vi "3a - QDSM message.vi"() -> ()   [LabVIEW 2015]
uses:
  State/Parent Actor.lvclass
  Child Actor/Child Actor.lvclass
panel:
  in  "Choose Actor":bool
  out "On Off Indicator":bool
  out "Dirrection indicator":enum16{"Forward", "Reverse"}(ring)
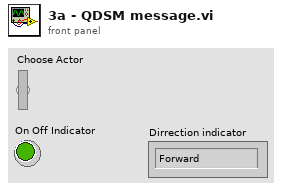
[diagram p1: front panel]
types:
  T1 = cluster{"Command":string, "Data":enum16{"Forward", "Reverse"}}
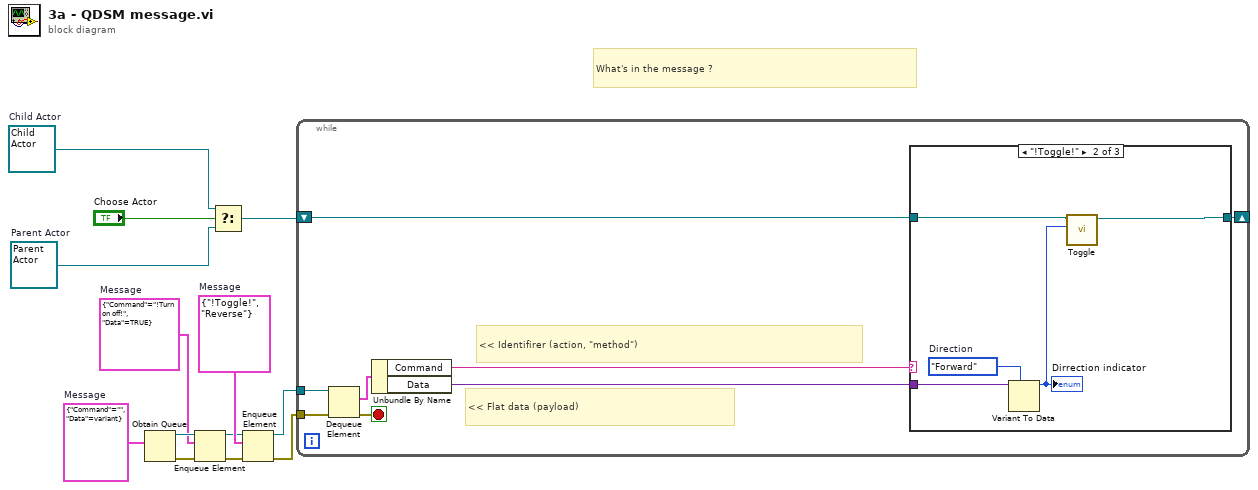
[diagram p0: block diagram]
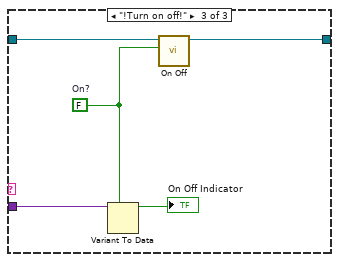
[diagram p3: hidden frame]
diagram:
  w2 = refnum<class "Child Actor.lvclass"> refnum  # Child Actor
  w4 = refnum<class "Parent Actor.lvclass"> refnum  # Parent Actor
  w5 = cluster{"Command":string, "Data":bool} {"Command"="!Turn on off!", "Data"=TRUE}  # Message
  w12 = T1 {"Command"="!Toggle!", "Data"=enum."Reverse"}  # Message
  w13 = cluster{"Command":string, "Data":variant} {"Command"="", "Data"=variant}  # Message
  # "What's in the message ?"
  n1 = Obtain Queue(element data type=w13) -> (queue out=w7:refnum<queue>, error out=w9:errorcluster)  [unwired: 4 in, 1 out]
  n2 = Enqueue Element(queue=w7, element=w5, error in (no error)=w9) -> (queue out=w6:refnum<queue>, error out=w8:errorcluster)  [unwired: 1 in, 1 out]
  n3 = Select(t=w2, s="Choose Actor", f=w4) -> (s? t:f=w3:refnum<class "Parent Actor.lvclass">)
  n4 = Enqueue Element(queue=w6, element=w12, error in (no error)=w8) -> (queue out=w10:refnum<queue>, error out=w11:errorcluster)  [unwired: 1 in, 1 out]
  n5 = while {
    tunnel: w11 -> [w21]
    tunnel: w10 -> [w20]
    shift-right: [w14] -> _
    shift-left: w3 -> [w15]
    stop <- w18 stop-if-true
    # "<< Flat data (payload)"
    # "<< Identifirer (action, \"method\")"
    n6 = Dequeue Element(queue=w20, error in (no error)=w21) -> (element=w19:cluster{"Command":string, "Data":variant}, error out=w18:errorcluster)  [unwired: 1 in, 2 out]
    n7 = Unbundle By Name(w19) -> ("Command"=w17:string, "Data"=w16:variant)
    n8 = case shown="\"!Toggle!\"" w17 {
      tunnel: w16 -> [_ w27 w32]
      tunnel: w15 -> [w22 w24 w31]
      tunnel: [w22 w23 w30] -> w14
      frame "", Default {
      }
      frame "!Toggle!" {
        w26 = enum16{"Forward", "Reverse"}."Forward"  # Direction
        n9 = Variant To Data(type=w26, Variant=w27) -> (data=w25:enum16{"Forward", "Reverse"})  [unwired: 1 in, 1 out]
        "Dirrection indicator" <- w25
        n10 = call-dynamic "Toggle.vi"("Dirrection"=w25, "State in"=w24) -> ("State out"=w23:refnum<class "Parent Actor.lvclass">)  [unwired: 8 in, 1 out]
      }
      frame "!Turn on off!" {
        w28 = FALSE  # On?
        n11 = Variant To Data(type=w28, Variant=w32) -> (data=→"On Off Indicator":bool)  [unwired: 1 in, 1 out]
        n12 = call-dynamic "On Off.vi"("On Off"=w28, "State in"=w31) -> ("State out"=w30:refnum<class "Parent Actor.lvclass">)  [unwired: 8 in, 1 out]
      }
    }
  }
